vi "Read child hwnd.vi"(8 "Error In":errorcluster, 11 "LV MDI.lvclass":refnum<class "LV MDI.lvclass">) -> (0 "Error Out":errorcluster, 2 "Child hWnd":u32, 3 "LV MDI.lvclass":refnum<class "LV MDI.lvclass">)   [LabVIEW 2016, in "LV MDI.lvclass"]
uses:
  LV MDI.lvclass
  LV MDI.lvclass/LV MDI.ctl
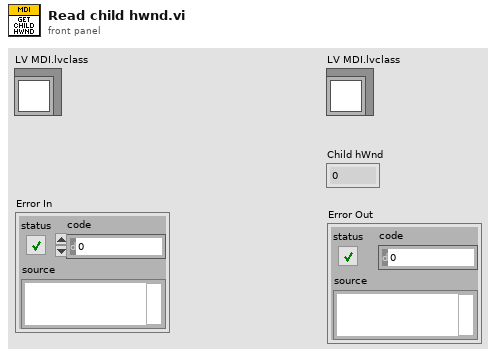
[diagram p1: front panel]
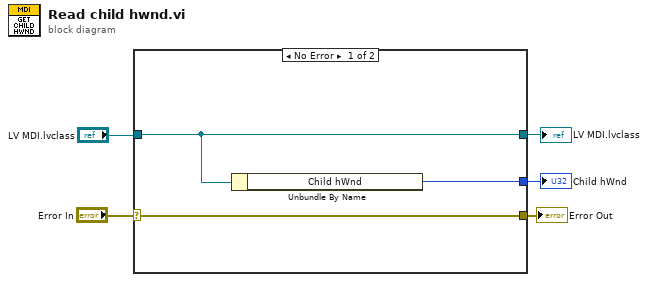
[diagram p0: block diagram]
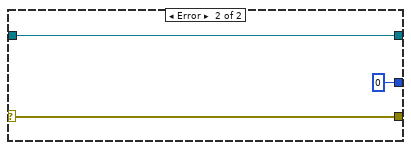
[diagram p2: hidden frame]
diagram:
  n1 = case shown="No Error" "Error In" {
    selector: "Error In" -> [w8 w11]
    tunnel: [w8 w11] -> w4
    tunnel: [w7 u32 0 ("Child hWnd")] -> w3
    tunnel: "LV MDI.lvclass" -> [w6 w9]
    tunnel: [w6 w9] -> w1
    frame No Error {
      n2 = Unbundle By Name(w6) -> ("Child hWnd"=w7:u32)
    }
    frame Error {
    }
  }
  "Error Out" <- w4
  "Child hWnd" <- w3
  "LV MDI.lvclass" <- w1
